vi "Ready to launch.vi"(8 "error in (no error)":errorcluster, 10 "GUID":string, 11 "Guardian in":refnum<class "Guardian.lvclass">) -> (0 "error out":errorcluster, 3 "Guardian out":refnum<class "Guardian.lvclass">)   [LabVIEW 2026, in "TALOS.lvlib" / "Guardian.lvlib" / "Guardian.lvclass"]
doc: "This VI checks that all the uServices that this Guardian should launch are up and running, and gives the entire list of uServices running back to who should check it (i.e. the Executor).\nNote that the uServices that are launched by another uService, and not from the Guardian, are given back in the list (the \"Ready to Launch?\" message will arrive also to them), but cannot be checked if they should run or not, because their launching is not Guardian responsibility (the Guardian responsibility is anyway to check if they're alive)."
uses:
  Guardian.lvclass
  C:/LabVIEW Code/TALOS/talos/Ancestor/Ancestor/Ancestor.lvclass
  Ancestor/Ancestor/Infinite Message Selector.ctl
  Support VIs/Go-NoGo.ctl
  Guardian.lvclass/Guardian.ctl
  Classes/uService List/uService List.lvclass/uService List.ctl
  Ancestor/Ancestor/Ancestor.lvclass/Ancestor.ctl
  Father of all uServices/Father of all uServices/Event Handler Items.ctl
  Classes/uService List/Get all IDs.vi
  Ancestor/Ancestor/Read ID.vi
  Support VIs/Generate Error.vi
  FGV/Error Memory/Get Error Description.vi
  Support VIs/Get PC name.vi
  Support VIs/Get Class Name.vi
  <vilib>/Utility/error.llb/Clear Errors.vi
  FGV/Error Memory/Error Memory Core.vi
  <vilib>/AdvancedString/Delimited String to 1D String Array.vi
  <vilib>/AdvancedString/Delimited String to 1D String Array (string).vi
  Support VIs/Circus Root Path.vi
  FGV/Error Memory/Error Crt Lvl checker.vi
  FGV/Error Memory/Error Memory Core.vi/40c8088d-b597-4017-91af-faa98e00292e.vi
  FGV/Error Memory/Error Memory Core.vi/d4a3ab98-063c-4e44-b43d-fbdcfe6c2be2.vi
  Support VIs/Global Constants.vi
  Support VIs/Global Memory.vi
  <vilib>/Utility/LVClass/Get LV Class Name.vi
  Support VIs/Is in Packed Library.vi
  Support VIs/TALOS Root path.vi
  Support VIs/Read CSV worksheet.vi
  <vilib>/Utility/error.llb/General Error Handler.vi
  Support VIs/Error Log.vi
  Ancestor/Ancestor/Ancestor.lvclass
  <vilib>/Comparison/Equal/Equal Functor/Equal Functor.lvclass
  Classes/uService List/uService List.lvclass
  TALOS.lvlib
  Father of all uServices/Father of all uServices/Father of all uServices.lvclass
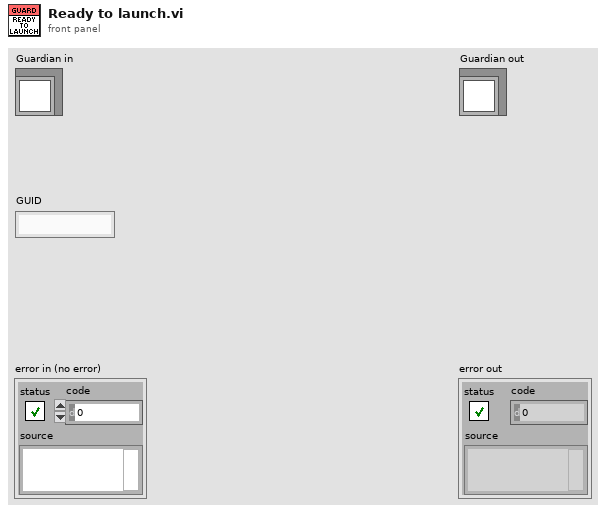
[diagram p1: front panel]
types:
  T1 = typedef "TALOS.lvlib/Ancestor.lvlib/Ancestor.lvclass/Infinite Message Selector.ctl" = enum16{"Start", "Stop", "Check", "Flush (Stop all)", "Init"}
  T2 = typedef "TALOS.lvlib/Go-NoGo.ctl" = cluster{"ID":string, "Status":bool, "Data":string[], "GUID":string}
  T3 = typedef "TALOS.lvlib/Father of all uServices.lvlib/Father of all uServices.lvclass/Event Handler Items.ctl" = enum16{"Button Pressed", "Message", "Ready to launch?", "Safe Mode", "Start RUN", "Stop RUN"}
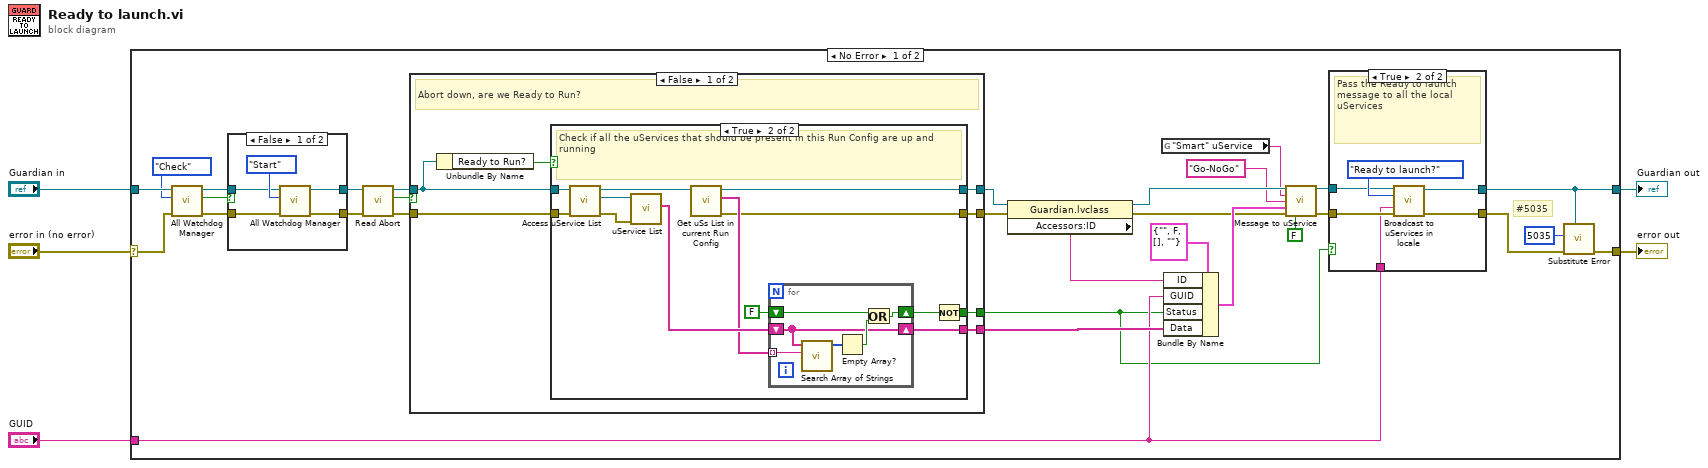
[diagram p0: block diagram]
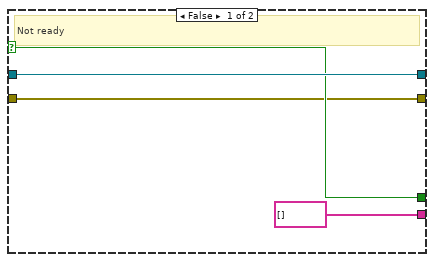
[diagram p3: hidden frame]
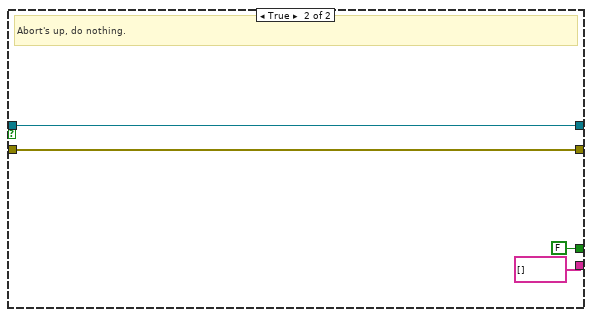
[diagram p4: hidden frame]
diagram:
  n1 = case shown="No Error" "error in (no error)" {
    selector: "error in (no error)" -> [w28 w86]
    tunnel: [w14 w86] -> w4
    tunnel: [w13 w85] -> w2
    tunnel: "Guardian in" -> [w29 w85]
    tunnel: "GUID" -> [w23 _]
    frame No Error {
      # "#5035"
      n2 = call "All Watchdog Manager.vi"("error in (no error)"=w28, "Infinite Message Selector"=Infinite_Message_Selector."Check", "Guardian in"=w29) -> ("error out"=w20:errorcluster, "Status"=w19:bool, "Guardian out"=w21:refnum<class "Guardian.lvclass">)  [unwired: 6 in]
      n3 = case shown="False" w19 {
        tunnel: w21 -> [w39 w42]
        tunnel: w20 -> [w38 w41]
        tunnel: [w37 w42] -> w11
        tunnel: [w36 w41] -> w10
        frame False {
          n4 = call "All Watchdog Manager.vi"("error in (no error)"=w38, "Infinite Message Selector"=Infinite_Message_Selector."Start", "Guardian in"=w39) -> ("error out"=w36:errorcluster, "Guardian out"=w37:refnum<class "Guardian.lvclass">)  [unwired: 6 in, 1 out]
        }
        frame True {
        }
      }
      n5 = call "Read Abort.vi"("error in (no error)"=w10, "Guardian in"=w11) -> ("error out"=w8:errorcluster, "Abort"=w7:bool, "Guardian out"=w9:refnum<class "Guardian.lvclass">)  [unwired: 7 in]
      n6 = case shown="False" w7 {
        tunnel: [w49 w75] -> w34
        tunnel: [w48 FALSE] -> w6
        tunnel: [w47 string[] [] ("All IDs")] -> w32
        tunnel: [w45 w76] -> w26
        tunnel: w9 -> [w44 w76]
        tunnel: w8 -> [w43 w75]
        frame False {
          # "Abort down, are we Ready to Run?"
          n7 = Unbundle By Name(w44) -> ("Ready to Run?"=w46:bool)
          n8 = case shown="True" w46 {
            selector: w46 -> [w52 _]
            tunnel: [w50 w54] -> w49
            tunnel: [w52 w64] -> w48
            tunnel: [string[] [] ("All IDs") w63] -> w47
            tunnel: w44 -> [w53 w58]
            tunnel: w43 -> [w50 w62]
            tunnel: [w53 w56] -> w45
            frame False {
              # "Not ready"
            }
            frame True {
              # "Check if all the uServices that should be present in this Run Config are up and running"
              n9 = call-dynamic "Access uService List.vi"("error in (no error)"=w62, "Ancestor in"=w58) -> ("error out"=w61:errorcluster, "uService List out"=w60:refnum<class "uService List.lvclass">, "Ancestor out"=w57:refnum<class "Guardian.lvclass">)  [unwired: 7 in]
              n10 = call-poly "uService List.vi"("error in (no error)"=w61, "uService List"=w60) -> ("All IDs"=w59:string[])  [unwired: 7 in, 2 out]
              n11 = call "Get uSs List in current Run Config.vi"("Guardian in"=w57) -> ("error out"=w54:errorcluster, "uSs in Run Config"=w55:string[], "Guardian out"=w56:refnum<class "Guardian.lvclass">)  [unwired: 8 in]
              n12 = for {
                tunnel: w55 -> [w72] mode=indexing
                shift-right: [w69] -> w65
                shift-left: FALSE -> [w68]
                shift-right: [w67] -> w63
                shift-left: w59 -> [w67]
                n13 = call "Search Array of Strings.vi"("search string"=w72, "Search array"=w67) -> ("indices"=w71:i32[])  [unwired: 8 in, 1 out]
                n14 = Empty Array?(array=w71) -> (empty?=w70:bool)
                n15 = Or(x=w68, y=w70) -> (x .or. y?=w69:bool)
              }
              n16 = Not(x=w65) -> (.not. x?=w64:bool)
            }
          }
        }
        frame True {
          # "Abort's up, do nothing."
        }
      }
      n17 = property class="Guardian.lvclass"(reference=w26, error in=w34) -> (reference out=w25:refnum<class "Guardian.lvclass">, error out=w33:errorcluster, "Accessors:ID"=w24:string)
      n18 = global read "Global Constants.vi" "\"Smart\" uService"() -> (w17:string)
      n19 = Bundle By Name(cluster=T2 {"ID"="", "Status"=FALSE, "Data"=[], "GUID"=""} ("Go-NoGo"), "ID"=w24, "GUID"=w23, "Status"=w6, "Data"=w32) -> (w35:T2)
      n20 = call "Message to uService.vi"("Guardian in"=w25, "uService ID"=w17, "Message"="Go-NoGo", "Data"=w35, "error in (no error)"=w33, "Locale?"=FALSE) -> ("Guardian out"=w27:refnum<class "Guardian.lvclass">, "error out"=w31:errorcluster)  [unwired: 8 in]
      n21 = case shown="True" w6 {
        tunnel: w31 -> [w77 w84]
        tunnel: w27 -> [w78 w82]
        tunnel: w23 -> [_ w81]
        tunnel: [w77 w80] -> w15
        tunnel: [w78 w79] -> w13
        frame False {
          # "Not ready for running."
        }
        frame True {
          # "Pass the Ready to launch message to all the local uServices"
          n22 = call "Broadcast to uServices in locale.vi"("Guardian in"=w82, "Event type"=Event_Handler_Items."Ready to launch?", "Data"=w81, "error in (no error)"=w84) -> ("Guardian out"=w79:refnum<class "Guardian.lvclass">, "error out"=w80:errorcluster)  [unwired: 10 in]
        }
      }
      n23 = call "Substitute Error.vi"("LabVIEW Object"=w13, "error in (no error)"=w15, "Error Code"=5035) -> ("error out"=w14:errorcluster)  [unwired: 8 in]
    }
    frame Error {
      # "Not doing anything here: if no reply from this Guardian is heard, sooner or later the Timeout for RUN! will expire."
    }
  }
  "error out" <- w4
  "Guardian out" <- w2
